vi "clear last element.vi"(8 "error in":errorcluster, 10 "Boolean Array":bool[](array[boolean]), 11 "ProXR in":refnum<class "ProXR.lvclass">) -> (0 "error out":errorcluster, 3 "ProXR out":refnum<class "ProXR.lvclass">)   [LabVIEW 2019, in "ProXR.lvlib" / "ProXR.lvclass"]
uses:
  Library/ProXR.lvclass
  C:/Users/Public/Documents/Development/builds/Instruments/DIG_IO.lvlibp/Library/DIG_IO.lvclass
  builds/Instruments/DIG_IO.lvlibp/Accessors/Read Channel Names.vi
  builds/Instruments/DIG_IO.lvlibp/Library/DIG_IO.lvclass
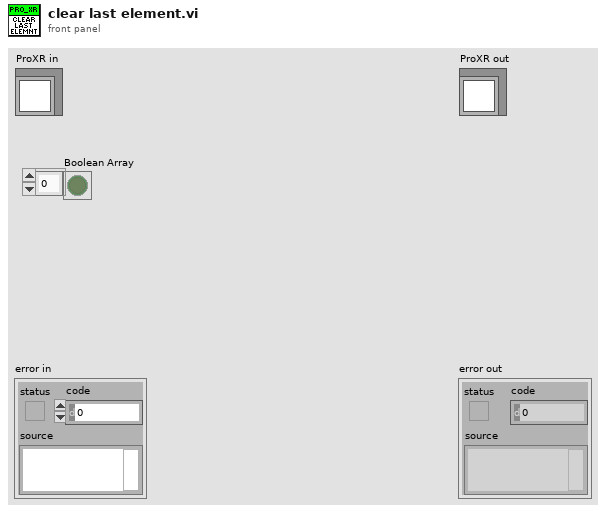
[diagram p1: front panel]
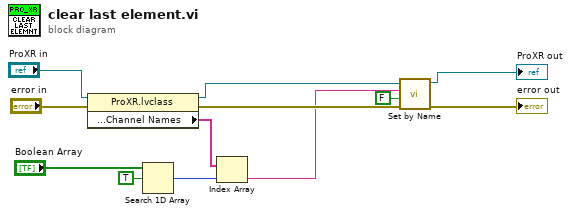
[diagram p0: block diagram]
diagram:
  n1 = property class="ProXR.lvclass"(reference="ProXR in", error in="error in") -> (reference out=w3:refnum<class "ProXR.lvclass">, error out=w6:errorcluster, "Accessors:Channel:Channel Names"=w8:string[])
  n2 = Search 1D Array(1D array="Boolean Array", element=TRUE) -> (index of element=w7:i32)  [unwired: 1 in]
  n3 = Index Array(array=w8, index=w7) -> (element=w5:string)
  n4 = call "Set by Name.vi"("error in"=w6, "Value"=FALSE, "Channel Name"=w5, "DIG_IO in"=w3) -> ("error out"=→"error out":errorcluster, "DIG_IO out"=→"ProXR out":refnum<class "ProXR.lvclass">)  [unwired: 6 in]
